vi "Get System Aliases.vi"() -> (1 "Number of INST":u32, 2 "Equipment Response":string[](array[string]), 3 "find list":string[](array[string]))   [LabVIEW 2019]
uses:
  <vilib>/Instr/_visa.llb/VISA Find Search Mode.ctl
  <vilib>/Instr/_visa.llb/VISA Configure Serial Port (Instr).vi
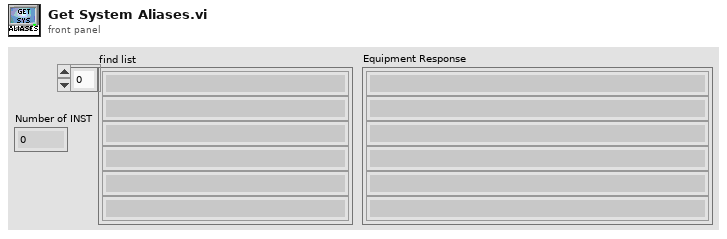
[diagram p1: front panel]
types:
  T1 = typedef "VISA Find Search Mode.ctl" = u32
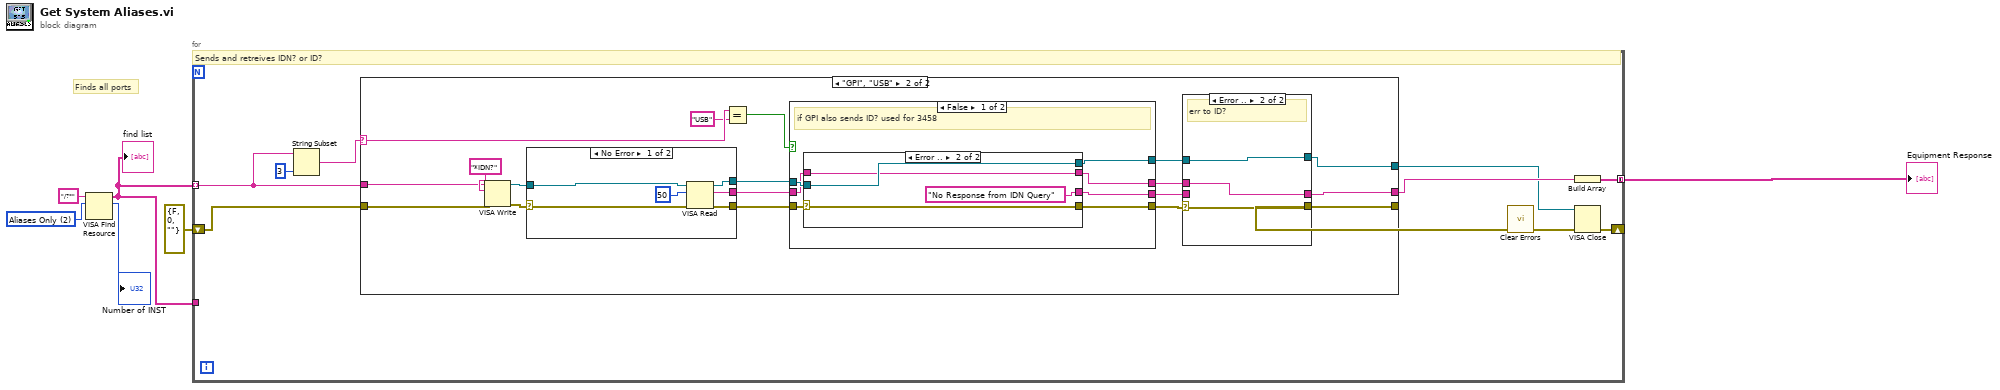
[diagram p0: block diagram]
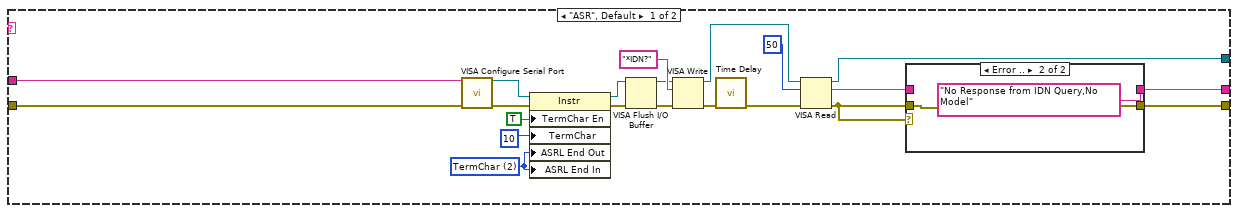
[diagram p2: hidden frame]
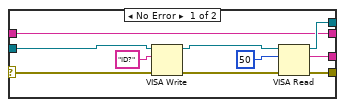
[diagram p5: hidden frame]
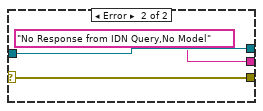
[diagram p7: hidden frame]
diagram:
  w4 = T1 2 items=["Canonical Names Only"=0, "Aliases Only"=2, "Include Matching Aliases"=3, "Include All Aliases"=4] ("Search Mode")
  # "Finds all ports"
  n1 = VISA Find Resource(10:w4, 11:"/?*" ("expression (\"?*\")")) -> (2:→"Number of INST":u32, 3:w1:string[])  [unwired: 1 in, 1 out]
  "find list" <- w1
  n2 = for {
    tunnel: w1 -> [w10] mode=indexing
    tunnel: [w16] -> w6 mode=concatenating
    tunnel: w1 -> [_]
    shift-right: [w14] -> _
    shift-left: errorcluster {"status"=FALSE, "code"=0, "source"=""} ("error out") -> [w12]
    # "Sends and retreives IDN? or ID?"
    n3 = String Subset(string=w10, length (rest)=3 ("length (rest)")) -> (substring=w8:string)  [unwired: 1 in]
    n4 = case shown="\"GPI\", \"USB\"" w8 {
      selector: w8 -> [_ w55]
      tunnel: [w21 w49] -> w13
      tunnel: [w22 w44] -> w7
      tunnel: w12 -> [w18 w42]
      tunnel: [w20 w51] -> w11
      tunnel: w10 -> [w19 w43]
      frame "ASR", Default {
        w17 = u16 2 items=["None", "Last Bit", "TermChar"] ("Serial Settings:End Mode for Reads")
        n5 = call-poly "VISA Configure Serial Port"("VISA resource name"=w19, "error in (no error)"=w18) -> ("VISA resource name out"=w28:refnum<visa-resource-name>, "error out"=w24:errorcluster)  [unwired: 12 in]
        n6 = property class="Instr"(reference=w28, error in=w24, "TermChar En"=TRUE ("Message Based Settings:Termination Character Enable"), "TermChar"=u8 10 ("Message Based Settings:Termination Character"), "ASRL End Out"=w17, "ASRL End In"=w17) -> (reference out=w29:refnum<visa-resource-name>, error out=w27:errorcluster)
        n7 = VISA Flush I/O Buffer(VISA resource name=w29, error in (no error)=w27) -> (VISA resource name out=w34:refnum<visa-resource-name>, error out=w23:errorcluster)  [unwired: 1 in]
        n8 = VISA Write(VISA resource name=w34, write buffer="*IDN?", error in (no error)=w23) -> (VISA resource name out=w36:refnum<visa-resource-name>, error out=w35:errorcluster)  [unwired: 1 out]
        n9 = call "Time Delay"("error in (no error)"=w35) -> ("error out"=w33:errorcluster)  [unwired: 10 in]
        n10 = VISA Read(VISA resource name=w36, byte count=u32 50, error in (no error)=w33) -> (VISA resource name out=w22:refnum<visa-resource-name>, read buffer=w30:string, error out=w31:errorcluster)  [unwired: 1 out]
        n11 = case shown="Error .." w31 {
          tunnel: w31 -> [w39 w41]
          tunnel: [w39 w41] -> w20
          tunnel: w30 -> [w38 _]
          tunnel: [w38 "No Response from IDN Query,No Model" ("read buffer")] -> w21
          frame No Error {
          }
          frame Error {
          }
        }
      }
      frame "GPI", "USB" {
        n12 = VISA Write(VISA resource name=w43, write buffer="*IDN?", error in (no error)=w42) -> (VISA resource name out=w46:refnum<visa-resource-name>, error out=w45:errorcluster)  [unwired: 1 out]
        n13 = case shown="No Error" w45 {
          selector: w45 -> [w90 w97]
          tunnel: w46 -> [w95 w98]
          tunnel: [w94 w98] -> w58
          tunnel: [w93 "No Response from IDN Query,No Model" ("read buffer")] -> w56
          tunnel: [w92 w97] -> w57
          frame No Error {
            n14 = VISA Read(VISA resource name=w95, byte count=u32 50, error in (no error)=w90) -> (VISA resource name out=w94:refnum<visa-resource-name>, read buffer=w93:string, error out=w92:errorcluster)  [unwired: 1 out]
          }
          frame Error {
          }
        }
        n15 = Equal?(x=w55, y="USB") -> (x = y?=w53:bool)
        n16 = case shown="False" w53 {
          tunnel: w58 -> [w72 w88]
          tunnel: w57 -> [w71 w89]
          tunnel: w56 -> [w70 w87]
          tunnel: [w69 w88] -> w52
          tunnel: [w68 w89] -> w50
          tunnel: [w67 w87] -> w47
          tunnel: [w66 w87] -> w48
          frame False {
            # "if GPI also sends ID? used for 3458"
            n17 = case shown="Error .." w71 {
              selector: w71 -> [w74 w84]
              tunnel: w72 -> [w81 w86]
              tunnel: [w75 w86] -> w69
              tunnel: [w76 "No Response from IDN Query" ("read buffer")] -> w66
              tunnel: w70 -> [w73 w83]
              tunnel: [w77 w84] -> w68
              tunnel: [w73 w83] -> w67
              frame No Error {
                n18 = VISA Write(VISA resource name=w81, write buffer="ID?", error in (no error)=w74) -> (VISA resource name out=w79:refnum<visa-resource-name>, error out=w78:errorcluster)  [unwired: 1 out]
                n19 = VISA Read(VISA resource name=w79, byte count=u32 50, error in (no error)=w78) -> (VISA resource name out=w75:refnum<visa-resource-name>, read buffer=w76:string, error out=w77:errorcluster)  [unwired: 1 out]
              }
              frame Error {
              }
            }
          }
          frame True {
            # "If USB device sends IDN? right thru"
          }
        }
        n20 = case shown="Error .." w50 {
          selector: w50 -> [w60 w63]
          tunnel: [w62 w65] -> w44
          tunnel: w52 -> [w62 w65]
          tunnel: [w60 w63] -> w51
          tunnel: [w61 w64] -> w49
          tunnel: w48 -> [w61 _]
          tunnel: w47 -> [_ w64]
          frame No Error {
            # "sends ID? reply"
          }
          frame Error {
            # "err to ID?"
          }
        }
      }
    }
    n21 = call <vilib>:"Clear Errors.vi"("error in (no error)"=w11) -> ("error out"=w15:errorcluster)  [unwired: 5 in, 1 out]
    n22 = Build Array(w13) -> (w16:string[])
    n23 = VISA Close(VISA resource name=w7, error in (no error)=w15) -> (error out=w14:errorcluster)
  }
  "Equipment Response" <- w6
